vi "PIDmain function.vi"() -> ()   [LabVIEW 2012]
uses:
  <vilib>/express/express arith-compare/Formula/XNode/ExpressFormulaBlockNode.xnode
  <vilib>/Analysis/NI_AALPro.lvlib
panel:
  in  "选择输入函数":enum16{"240sin(t)", "340sqrt(t)"}(ring)
  out "波形图表":dbl(graph)
  in  "请输入姓名":string="huang"
  in  "停止按钮":bool
  out "报警指示灯":bool=TRUE
  in  "KD":dbl=2.0
  in  "Ki":dbl=0.01
  in  "KP":dbl=1.0
  in  "水罐总高度h,单位cm":dbl=100.0
  in  "横截面积A,单位cm^2":dbl=20.0
  in  "h设定数值(60%-70%)":dbl=60.0 min=60.0 max=70.0
  in  "h最初数值，单位cm":dbl=50.0 min=0.0 max=100.0
  in  "PID调节，范围0-0.25A":sgl min=0 max=0.25
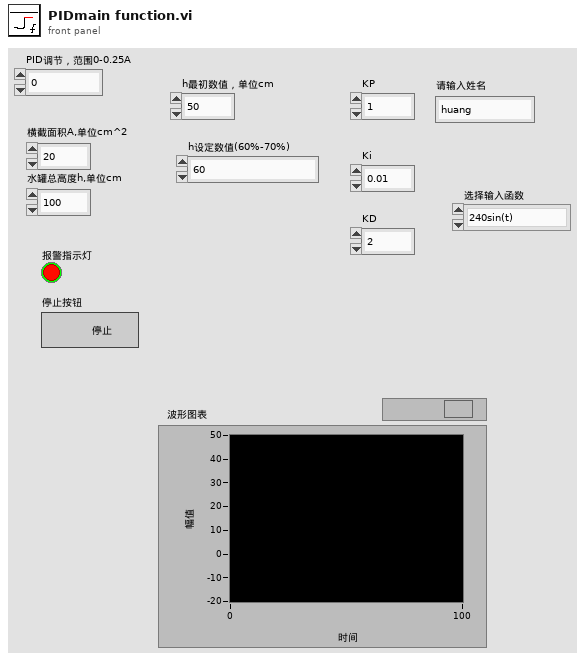
[diagram p1: front panel]
types:
  T1 = enum16{"open", "replace", "create", "open or create", "replace or create", "replace or create with confirmation"}
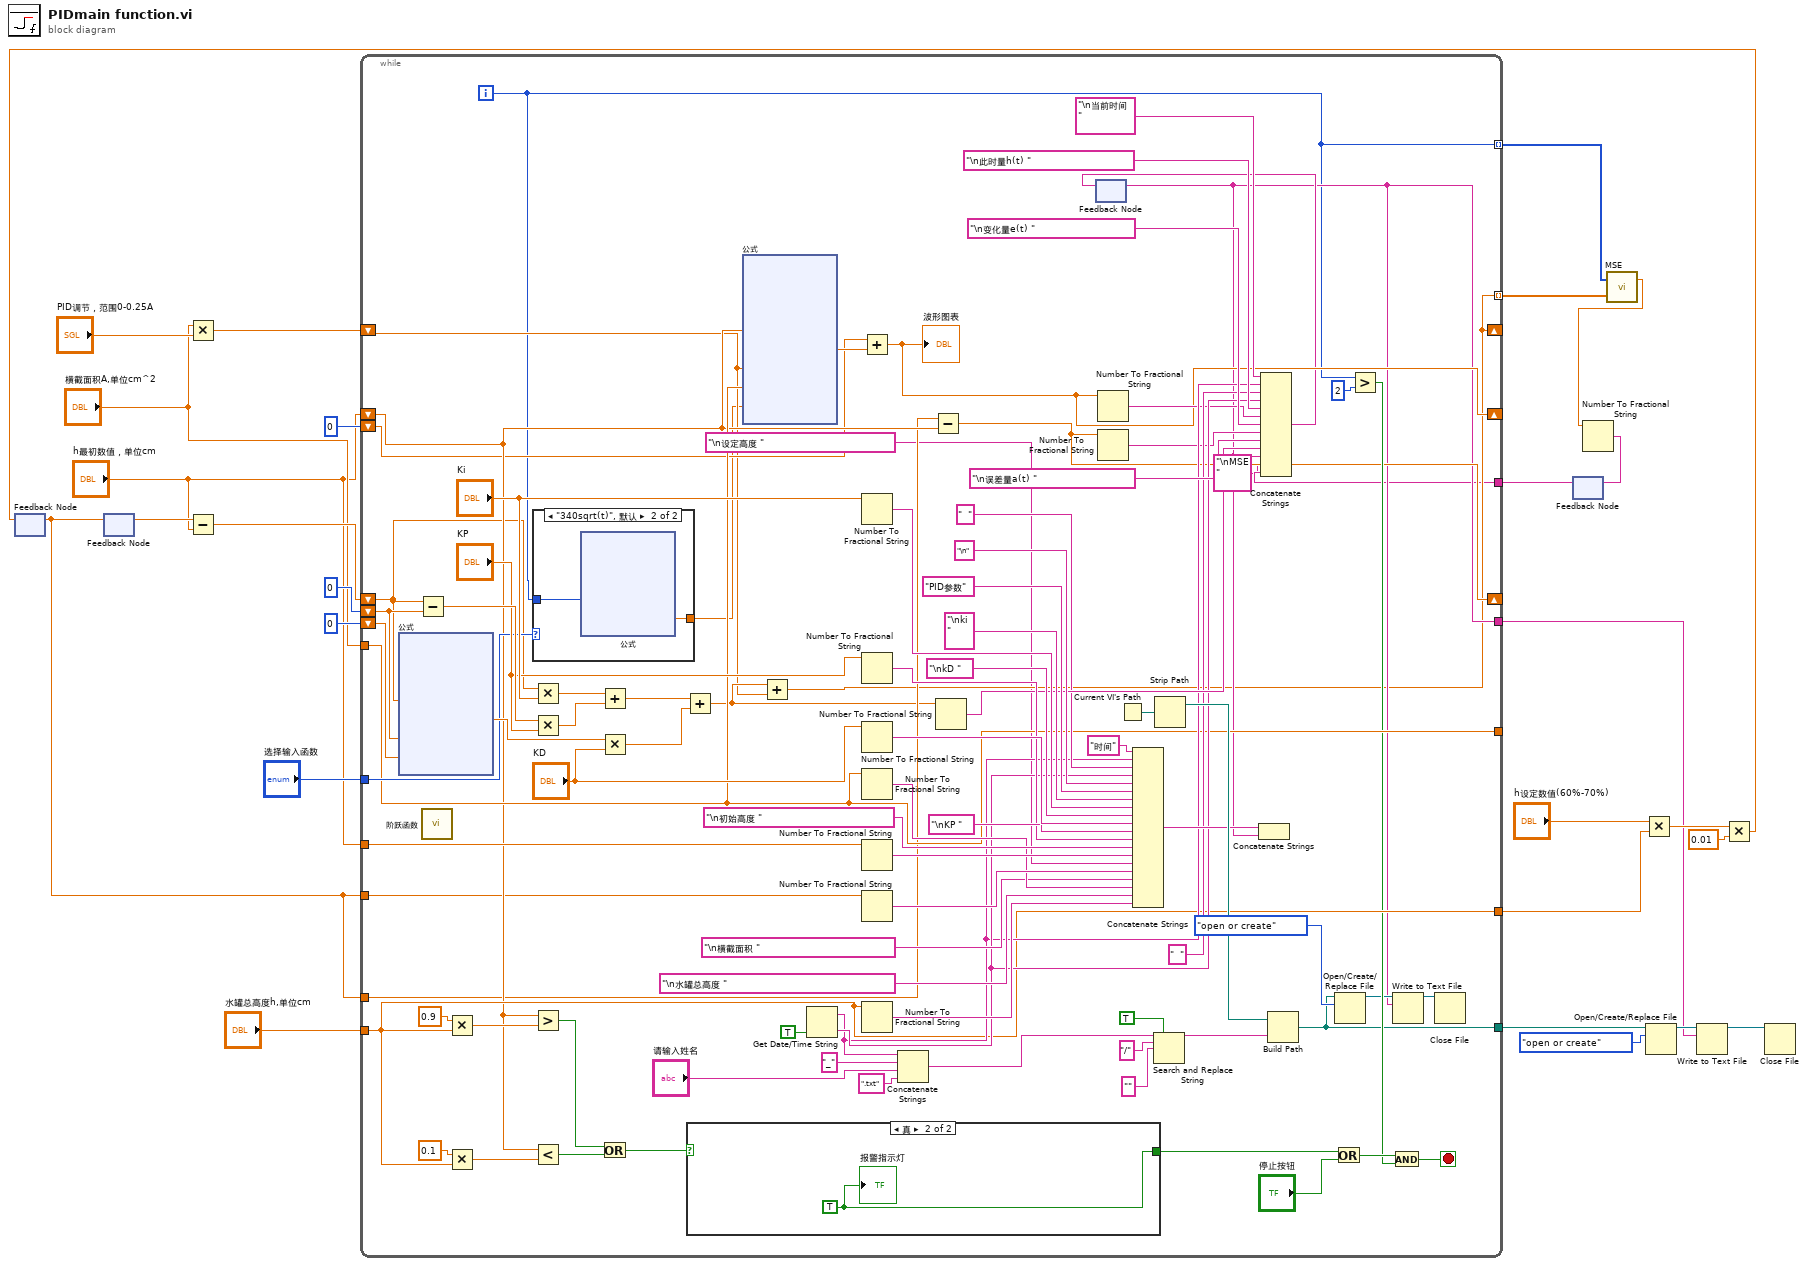
[diagram p0: block diagram]
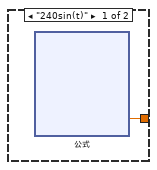
[diagram p2: hidden frame]
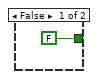
[diagram p3: hidden frame]
diagram:
  n1 = feedback #1() -> (w11:dbl)  [unwired: 1 in]
  n2 = feedback-in #2(w11) -> ()
  n3 = feedback #2() -> (w15:dbl)  [unwired: 1 in]
  n4 = Multiply(x="横截面积A,单位cm^2", y="PID调节，范围0-0.25A") -> (x*y=w17:dbl)
  n5 = Subtract(x=w15, y="h最初数值，单位cm") -> (x-y=w26:dbl)
  n6 = feedback #3() -> (w1:string)  [unwired: 1 in]
  n7 = while {
    shift-right: [w38] -> _
    shift-left: "h最初数值，单位cm" -> [w51]
    shift-left: 0 -> [w48]
    shift-right: [w39] -> _
    shift-left: w26 -> [w36]
    shift-left: 0 -> [w103]
    shift-left: 0 -> [w102]
    tunnel: "h最初数值，单位cm" -> [w85]
    tunnel: [w58] -> w23
    tunnel: "选择输入函数" -> [w71]
    tunnel: [w57] -> _
    tunnel: "水罐总高度h,单位cm" -> [w58]
    tunnel: "横截面积A,单位cm^2" -> [w57]
    shift-right: [w33] -> _
    shift-left: w17 -> [w45]
    tunnel: w11 -> [w49]
    tunnel: w11 -> [w47]
    tunnel: [w35] -> w7
    tunnel: [w34] -> w6
    tunnel: [w33] -> w5 mode=indexing
    tunnel: [w30] -> w4 mode=indexing
    tunnel: w1 -> [w32]
    i -> [w30]
    stop <- w54 stop-if-true
    n8 = xnode "公式"("e1"=w36, "e2"=w103, "e3"=w102) -> ("结果"=w101:dbl)  [unwired: 1 in, 1 out]
    n9 = Subtract(x=w36, y=w103) -> (x-y=w100:dbl)
    n10 = call "阶跃函数.vi"() -> ()  [unwired: 1 in, 1 out]
    n11 = Multiply(x=0.9 ("KD 2"), y=w58) -> (x*y=w53:dbl)
    n12 = Multiply(x=0.1 ("KD 2"), y=w58) -> (x*y=w52:dbl)
    n13 = case shown="\"340sqrt(t)\", 默认" w71 {
      tunnel: [w117 w127] -> w29
      tunnel: w30 -> [_ w126]
      frame "240sin(t)" {
        n14 = xnode "公式"() -> ("结果"=w117:dbl)  [unwired: 2 in, 1 out]
      }
      frame "340sqrt(t)", Default {
        n15 = xnode "公式"("t"=w126) -> ("结果"=w127:dbl)  [unwired: 1 in, 1 out]
      }
    }
    n16 = Multiply(x=w36, y="Ki") -> (x*y=w99:dbl)
    n17 = Multiply(x=w100, y="KP") -> (x*y=w98:dbl)
    n18 = Greater?(x=w51, y=w53) -> (0:w116:bool)
    n19 = Less?(x=w51, y=w52) -> (x < y?=w115:bool)
    n20 = Add(x=w99, y=w98) -> (x+y=w97:dbl)
    n21 = Multiply(x=w101, y="KD") -> (x*y=w96:dbl)
    n22 = Or(x=w116, y=w115) -> (x .or. y?=w114:bool)
    n23 = Add(x=w97, y=w96) -> (x+y=w46:dbl)
    n24 = case shown="真" w114 {
      tunnel: [FALSE w163] -> w113
      frame False {
      }
      frame True {
        w163 = TRUE
        "报警指示灯" <- w163
      }
    }
    n25 = xnode "公式"("h"=w51, "a"=w45, "A"=w57, "f"=w29) -> ("结果"=w50:dbl)  [unwired: 1 in, 1 out]
    n26 = Add(x=w46, y=w45) -> (x+y=w33:dbl)
    n27 = Get Date/Time String(want seconds? (F)=TRUE ("需要秒？(F)")) -> (date string=w61:string, time string=w62:string)  [unwired: 2 in]
    n28 = Add(x=w48, y=w50) -> (x+y=w38:dbl)
    "波形图表" <- w38
    n29 = Number To Fractional String(number="Ki") -> (F-format string=w91:string)  [unwired: 3 in]
    n30 = Number To Fractional String(number="KP") -> (F-format string=w78:string)  [unwired: 3 in]
    n31 = Number To Fractional String(number="KD") -> (F-format string=w90:string)  [unwired: 3 in]
    n32 = Number To Fractional String(number=w57) -> (F-format string=w82:string)  [unwired: 3 in]
    n33 = Number To Fractional String(number=w85) -> (F-format string=w84:string)  [unwired: 3 in]
    n34 = Number To Fractional String(number=w49) -> (F-format string=w83:string)  [unwired: 3 in]
    n35 = Number To Fractional String(number=w58) -> (F-format string=w79:string)  [unwired: 3 in]
    n36 = Concatenate Strings(w61, "_" ("字符串"), "请输入姓名", ".txt" ("名称或相对路径")) -> (w74:string)
    n37 = Subtract(x=w47, y=w51) -> (x-y=w39:dbl)
    n38 = Number To Fractional String(number=w46) -> (F-format string=w67:string)  [unwired: 3 in]
    n39 = feedback #4() -> (w35:string)  [unwired: 1 in]
    n40 = Number To Fractional String(number=w38) -> (F-format string=w40:string)  [unwired: 3 in]
    n41 = Number To Fractional String(number=w39) -> (F-format string=w41:string)  [unwired: 3 in]
    n42 = Current VI's Path() -> (path=w108:path)
    n43 = Concatenate Strings("时间" ("字符串"), w61, "  " ("字符串"), w62, "\n" ("字符串"), "PID参数" ("字符串"), "\nki " ("字符串"), w91, "\nkD " ("字符串"), w90, "\nKP " ("字符串"), w78, "\n初始高度 " ("字符串"), w84, "\n设定高度 " ("字符串"), w83, "\n横截面积 " ("字符串"), w82, "\n水罐总高度 " ("字符串"), w79) -> (w70:string)
    n44 = Search and Replace String(replace all?=TRUE ("替换全部？(F)"), input string=w74, search string="/" ("搜索字符串"), replace string="" ("替换字符串(\"\")")) -> (result string=w73:string)  [unwired: 4 in, 3 out]
    n45 = Strip Path(path=w108) -> (stripped path=w106:path)  [unwired: 1 out]
    n46 = Concatenate Strings(w70, w35) -> ()  [unwired: 1 out]
    n47 = Concatenate Strings("\n当前时间 " ("字符串"), w61, "  " ("字符串"), w62, "\n此时量h(t) " ("字符串"), w40, "\n变化量e(t) " ("字符串"), w41, "\n误差量a(t) " ("字符串"), w67, w35, "\nMSE " ("字符串"), w32) -> (w37:string)
    n48 = feedback-in #4(w37) -> ()
    n49 = Build Path(base path=w106, name or relative path=w73) -> (appended path=w34:path)
    n50 = Or(x=w113, y="停止按钮") -> (x .or. y?=w56:bool)
    n51 = Open/Create/Replace File(file path (use dialog)=w34, operation (0:open)=T1."open or create" ("操作(0:open)")) -> (refnum out=w42:refnum<file>)  [unwired: 4 in, 2 out]
    n52 = Greater?(x=w30, y=2) -> (0:w55:bool)
    n53 = And(x=w56, y=w55) -> (x .and. y?=w54:bool)
    n54 = Write to Text File(file (use dialog)=w42, text=w35) -> (refnum out=w43:refnum<file>)  [unwired: 2 in, 2 out]
    n55 = Close File(refnum=w43) -> ()  [unwired: 1 in, 2 out]
  }
  n56 = call <vilib>:"MSE.vi"("X Values"=w5, "Y Values"=w4) -> ("mse"=w3:dbl)  [unwired: 1 out]
  n57 = Number To Fractional String(number=w3) -> (F-format string=w2:string)  [unwired: 3 in]
  n58 = feedback-in #3(w2) -> ()
  n59 = Multiply(x="h设定数值(60%-70%)", y=w23) -> (x*y=w21:dbl)
  n60 = Open/Create/Replace File(file path (use dialog)=w6, operation (0:open)=T1."open or create" ("操作(0:open)")) -> (refnum out=w8:refnum<file>)  [unwired: 4 in, 2 out]
  n61 = Write to Text File(file (use dialog)=w8, text=w7) -> (refnum out=w9:refnum<file>)  [unwired: 2 in, 2 out]
  n62 = Multiply(x=w21, y=0.01) -> (x*y=w14:dbl)
  n63 = feedback-in #1(w14) -> ()
  n64 = Close File(refnum=w9) -> ()  [unwired: 1 in, 2 out]
